vi "Cache Previous Values.vi"(8 "error in (no error)":errorcluster, 11 "2WayValve in":refnum<class "2WayValveH.lvclass">) -> (0 "error out":errorcluster, 3 "2WayValve out":refnum<class "2WayValveH.lvclass">)   [LabVIEW 2020, in "VolatusGUIElements.lvlib" / "2WayValveH.lvclass"]
uses:
  2WayValveH.lvclass
  2WayValveH.lvclass/2WayValveH.ctl
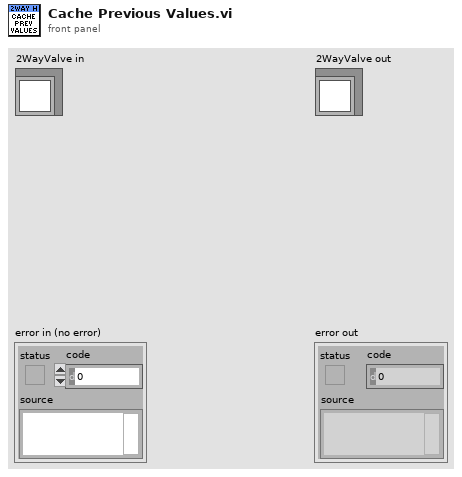
[diagram p1: front panel]
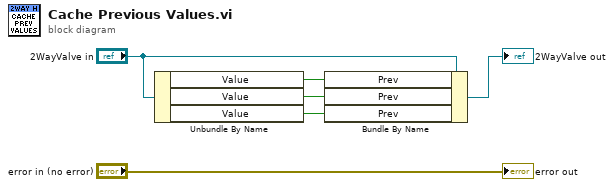
[diagram p0: block diagram]
diagram:
  n1 = Unbundle By Name("2WayValve in") -> ("Value"=w3:bool, "Value"=w2:bool, "Value"=w1:bool)
  n2 = Bundle By Name(cluster="2WayValve in", "Prev"=w3, "Prev"=w2, "Prev"=w1) -> (→"2WayValve out":refnum<class "2WayValveH.lvclass">)
  "error out" <- "error in (no error)"
